vi "r1y.vi"   [LabVIEW 2019]
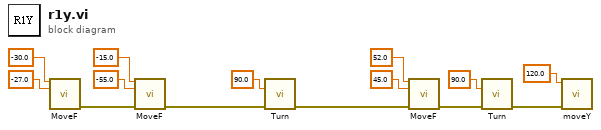
[diagram p0: block diagram]
diagram:
  n1 = call "MoveF.vi"("X"=-30.0, "Y"=-27.0) -> ("error out"=w5:errorcluster)  [unwired: 13 in]
  n2 = call "MoveF.vi"("X"=-15.0, "Y"=-55.0, "error in (no error)"=w5) -> ("error out"=w7:errorcluster)  [unwired: 12 in]
  n3 = call "Turn.vi"("¨¤«×"=90.0, "error in (no error)"=w7) -> ("error out"=w10:errorcluster)  [unwired: 13 in]
  n4 = call "MoveF.vi"("X"=52.0, "Y"=45.0, "error in (no error)"=w10) -> ("error out"=w12:errorcluster)  [unwired: 12 in]
  n5 = call "Turn.vi"("¨¤«×"=90.0, "error in (no error)"=w12) -> ("error out"=w14:errorcluster)  [unwired: 13 in]
  n6 = call "moveY.vi"("error in (no error)"=w14, "Y"=120.0) -> ()  [unwired: 9 in, 1 out]
